vi "PhasorROI2IMG.vi"(0 "Intensity":dbl[][](array[numeric]), 1 "Auto Scale?":bool, 2 "Threshold (max)":dbl, 3 "Threshold (min)":dbl, 4 "G Data":dbl[][](array[numeric]), 5 "S Data":dbl[][](array[numeric]), 6 "Pic Reference":refnum<vi>, 7 "ROI? array":bool[](array[boolean]), 9 "Radius array":dbl[](array[numeric]), 11 "Center array":cluster{dbl, dbl}[](array[cluster]), 13 "Color array":u32[](array[numeric])) -> (14 "new picture":picture)   [LabVIEW 2018]
uses:
  <vilib>/picture/picture.llb/Draw True-Color Pixmap.vi
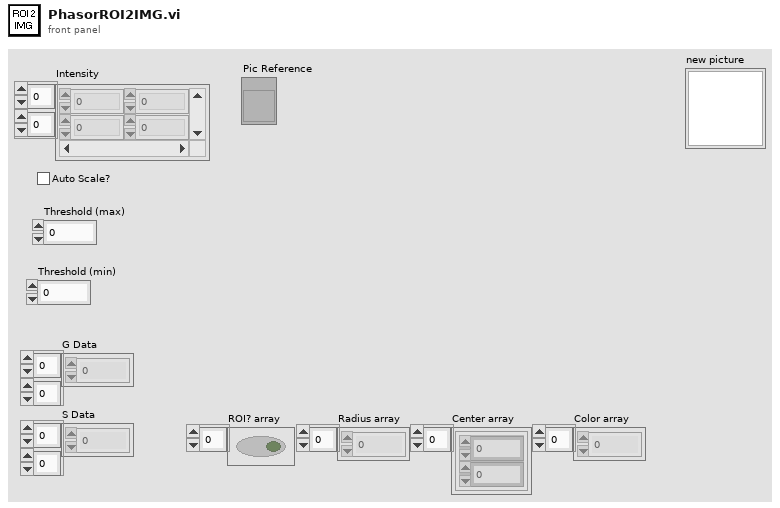
[diagram p1: front panel]
types:
  T1 = typedef "LVBoundsTypeDef.ctl" = cluster{"Width":u32, "Height":u32}
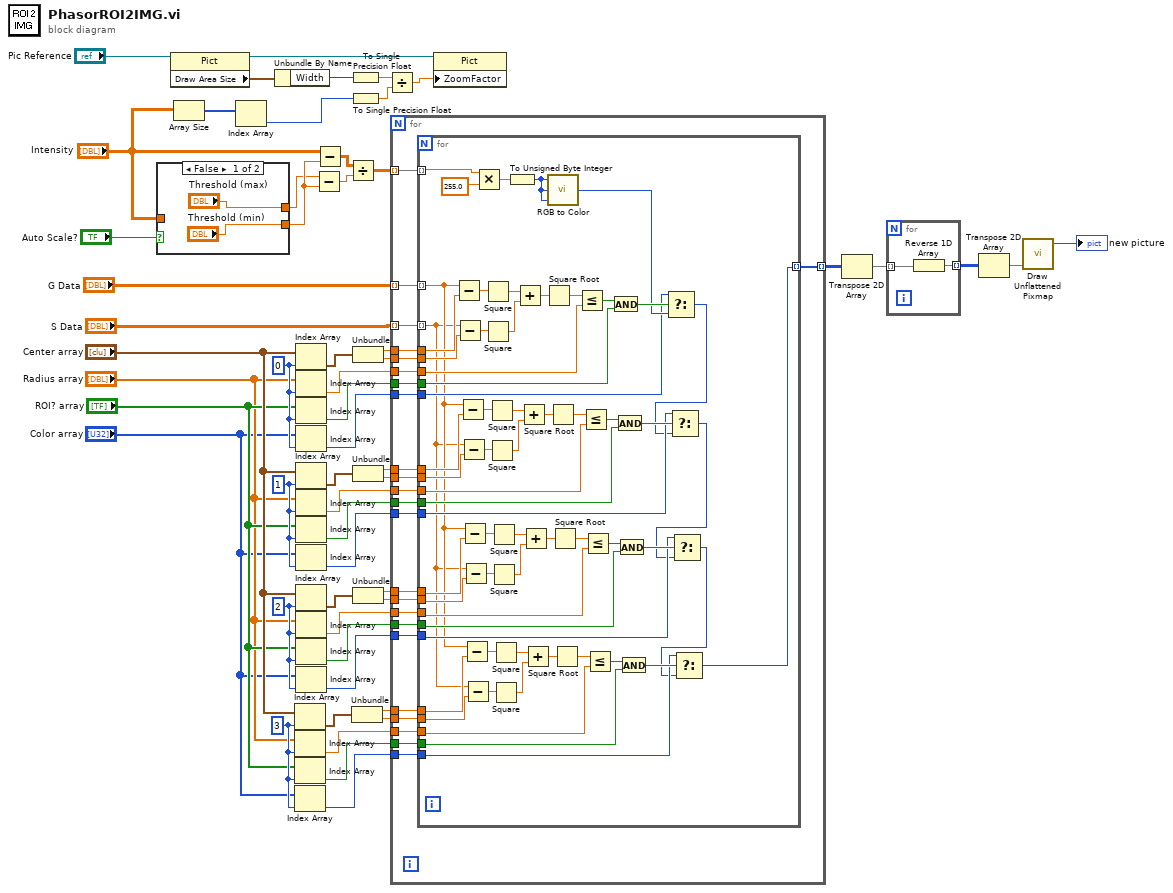
[diagram p0: block diagram]
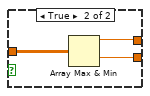
[diagram p2: hidden frame]
diagram:
  w7 = 3 ("index")
  w16 = 2 ("index")
  w21 = 1 ("index")
  w30 = 0 ("index")
  n1 = case shown="False" "Auto Scale?" {
    tunnel: "Intensity" -> [_ w60]
    tunnel: ["Threshold (max)" w59] -> w47
    tunnel: ["Threshold (min)" w58] -> w48
    frame False {
    }
    frame True {
      n2 = Array Max & Min(array=w60) -> (max value=w59:dbl, min value=w58:dbl)  [unwired: 2 out]
    }
  }
  n3 = property on="Property Node" class="Pict"(reference="Pic Reference") -> (reference out=w37:refnum<vi>, "Draw Area Size"=w39:T1)  [unwired: 1 in, 1 out]
  n4 = Array Size(array="Intensity") -> (size(s)=w35:i32[])
  n5 = Index Array(array=w35) -> (element=w34:i32)  [unwired: 1 in]
  n6 = Unbundle By Name(w39) -> ("Width"=w43:u32)
  n7 = Index Array(array="Center array", index=w7) -> (element=w8:cluster{dbl, dbl})
  n8 = Index Array(array="Radius array", index=w7) -> (element=w9:dbl)
  n9 = Index Array(array="ROI? array", index=w7) -> (element=w10:bool)
  n10 = Index Array(array="Color array", index=w7) -> (element=w11:u32)
  n11 = Index Array(array="Center array", index=w30) -> (element=w29:cluster{dbl, dbl})
  n12 = Index Array(array="Radius array", index=w30) -> (element=w28:dbl)
  n13 = Index Array(array="ROI? array", index=w30) -> (element=w27:bool)
  n14 = Index Array(array="Color array", index=w30) -> (element=w26:u32)
  n15 = Index Array(array="Center array", index=w21) -> (element=w22:cluster{dbl, dbl})
  n16 = Index Array(array="Radius array", index=w21) -> (element=w23:dbl)
  n17 = Index Array(array="ROI? array", index=w21) -> (element=w24:bool)
  n18 = Index Array(array="Color array", index=w21) -> (element=w25:u32)
  n19 = Index Array(array="Center array", index=w16) -> (element=w15:cluster{dbl, dbl})
  n20 = Index Array(array="Radius array", index=w16) -> (element=w14:dbl)
  n21 = Index Array(array="ROI? array", index=w16) -> (element=w13:bool)
  n22 = Index Array(array="Color array", index=w16) -> (element=w12:u32)
  n23 = Subtract(x=w47, y=w48) -> (x-y=w51:dbl)
  n24 = Subtract(x="Intensity", y=w48) -> (x-y=w50:dbl[][])
  n25 = Divide(x=w50, y=w51) -> (x/y=w32:dbl[][])
  n26 = To Single Precision Float(number=w43) -> (single precision float=w41:sgl)
  n27 = To Single Precision Float(number=w34) -> (single precision float=w42:sgl)
  n28 = Unbundle(w8) -> (w5:dbl, w6:dbl)
  n29 = Unbundle(w29) -> (w53:dbl, w52:dbl)
  n30 = Unbundle(w22) -> (w19:dbl, w20:dbl)
  n31 = Unbundle(w15) -> (w18:dbl, w17:dbl)
  n32 = Divide(x=w41, y=w42) -> (x/y=w38:sgl)
  n33 = for {
    tunnel: "G Data" -> [w84] mode=indexing
    tunnel: "S Data" -> [w83] mode=indexing
    tunnel: w53 -> [w82]
    tunnel: w52 -> [w81]
    tunnel: w28 -> [w80]
    tunnel: w32 -> [w79] mode=indexing
    tunnel: [w78] -> w31 mode=indexing
    tunnel: w27 -> [w77]
    tunnel: w26 -> [w76]
    tunnel: w19 -> [w71]
    tunnel: w20 -> [w72]
    tunnel: w23 -> [w73]
    tunnel: w24 -> [w74]
    tunnel: w25 -> [w75]
    tunnel: w18 -> [w70]
    tunnel: w17 -> [w69]
    tunnel: w14 -> [w68]
    tunnel: w13 -> [w67]
    tunnel: w12 -> [w66]
    tunnel: w5 -> [w61]
    tunnel: w6 -> [w62]
    tunnel: w9 -> [w63]
    tunnel: w10 -> [w64]
    tunnel: w11 -> [w65]
    n34 = for {
      tunnel: w84 -> [w90] mode=indexing
      tunnel: w83 -> [w89] mode=indexing
      tunnel: w82 -> [w147]
      tunnel: w81 -> [w146]
      tunnel: w80 -> [w145]
      tunnel: w79 -> [w135] mode=indexing
      tunnel: [w85] -> w78 mode=indexing
      tunnel: w77 -> [w133]
      tunnel: w76 -> [w130]
      tunnel: w71 -> [w121]
      tunnel: w72 -> [w120]
      tunnel: w73 -> [w119]
      tunnel: w74 -> [w118]
      tunnel: w75 -> [w117]
      tunnel: w70 -> [w100]
      tunnel: w69 -> [w99]
      tunnel: w68 -> [w98]
      tunnel: w67 -> [w97]
      tunnel: w66 -> [w96]
      tunnel: w61 -> [w95]
      tunnel: w62 -> [w94]
      tunnel: w63 -> [w93]
      tunnel: w64 -> [w92]
      tunnel: w65 -> [w91]
      # "Pixel Level"
      n35 = Subtract(x=w90, y=w147) -> (x-y=w144:dbl)
      n36 = Subtract(x=w89, y=w146) -> (x-y=w143:dbl)
      n37 = Subtract(x=w90, y=w121) -> (x-y=w122:dbl)
      n38 = Subtract(x=w89, y=w120) -> (x-y=w123:dbl)
      n39 = Subtract(x=w90, y=w100) -> (x-y=w116:dbl)
      n40 = Subtract(x=w89, y=w99) -> (x-y=w115:dbl)
      n41 = Subtract(x=w90, y=w95) -> (x-y=w101:dbl)
      n42 = Subtract(x=w89, y=w94) -> (x-y=w102:dbl)
      n43 = Multiply(x=w135, y=255.0) -> (x*y=w137:dbl)
      n44 = Square(x=w144) -> (x^2=w142:dbl)
      n45 = Square(x=w143) -> (x^2=w141:dbl)
      n46 = Square(x=w122) -> (x^2=w124:dbl)
      n47 = Square(x=w123) -> (x^2=w125:dbl)
      n48 = Square(x=w116) -> (x^2=w114:dbl)
      n49 = Square(x=w115) -> (x^2=w113:dbl)
      n50 = Square(x=w101) -> (x^2=w103:dbl)
      n51 = Square(x=w102) -> (x^2=w104:dbl)
      n52 = To Unsigned Byte Integer(number=w137) -> (unsigned 8bit integer=w138:u8)
      n53 = Add(x=w142, y=w141) -> (x+y=w140:dbl)
      n54 = Add(x=w124, y=w125) -> (x+y=w126:dbl)
      n55 = Add(x=w114, y=w113) -> (x+y=w112:dbl)
      n56 = Add(x=w103, y=w104) -> (x+y=w105:dbl)
      n57 = Square Root(x=w140) -> (sqrt(x)=w139:dbl)
      n58 = call <vilib>:"RGB to Color.vi"("B"=w138, "G"=w138, "R"=w138) -> ("Color"=w131:u32)
      n59 = Square Root(x=w126) -> (sqrt(x)=w127:dbl)
      n60 = Square Root(x=w112) -> (sqrt(x)=w111:dbl)
      n61 = Square Root(x=w105) -> (sqrt(x)=w106:dbl)
      n62 = Less Or Equal?(x=w139, y=w145) -> (x <= y?=w134:bool)
      n63 = Less Or Equal?(x=w127, y=w119) -> (x <= y?=w128:bool)
      n64 = Less Or Equal?(x=w111, y=w98) -> (x <= y?=w110:bool)
      n65 = Less Or Equal?(x=w106, y=w93) -> (x <= y?=w107:bool)
      n66 = And(x=w134, y=w133) -> (x .and. y?=w132:bool)
      n67 = And(x=w128, y=w118) -> (x .and. y?=w129:bool)
      n68 = And(x=w110, y=w97) -> (x .and. y?=w109:bool)
      n69 = And(x=w107, y=w92) -> (x .and. y?=w108:bool)
      n70 = Select(t=w130, s=w132, f=w131) -> (s? t:f=w88:u32)
      n71 = Select(t=w117, s=w129, f=w88) -> (s? t:f=w87:u32)
      n72 = Select(t=w96, s=w109, f=w87) -> (s? t:f=w86:u32)
      n73 = Select(t=w91, s=w108, f=w86) -> (s? t:f=w85:u32)
    }
  }
  n74 = property on="Property Node" class="Pict"(reference=w37, "ZoomFactor"=w38) -> ()  [unwired: 1 in, 2 out]
  n75 = Transpose 2D Array(2D array=w31) -> (transposed array=w46:u32[][])
  n76 = for {
    tunnel: w46 -> [w149] mode=indexing
    tunnel: [w148] -> w45 mode=indexing
    n77 = Reverse 1D Array(array=w149) -> (reversed array=w148:u32[])
  }
  n78 = Transpose 2D Array(2D array=w45) -> (transposed array=w44:u32[][])
  n79 = call-poly <vilib>:"Draw Unflattened Pixmap.vi"("data (RGB format)"=w44) -> ("new picture"=→"new picture":picture)  [unwired: 8 in]
